vi "Forebrain.vi"() -> ()   [LabVIEW 2012]
doc: "This VI contrains the Forebrain within the Olin Robot Architecture. It must be run first to load the appropriate mission definition files. It contains a finite state machine built around a tabbed Operator interface that will guide an operator through the startup, run shutdown mission sequence. After running it, run the Midbrain and Hindbrain VIS."
panel:
  in  "Lidar cutoff":dbl
  in  "behavior weights":i8[](array[numeric])=[0, 1, 0]
  in  "Follow right?":bool
  in  "Lider good scale mult":dbl=0.0125
  in  "Lider good scale add":dbl
  in  "Lider speed scale add":dbl
  in  "Lider speed scale mult":dbl=0.0175
  in  "IR scaling div":dbl=150.0
  in  "IR Following Distance":i32=300
  out "Ir distance":i16
  in  "Manual Override":bool=TRUE
  out "Send String for AutoMode":string="$B^"
  in  "Soft E-Stop":bool
  out "NXT String Received":string
  out "return count":u32
  out "error out":errorcluster
  in  "error in 2":errorcluster
  out "Desired \nVelocity":i16=5
  out "Local\nHeading":i16=90
  out "Ycurrent":dbl format="%#_3g"
  out "Xcurrent":dbl format="%#_3g"
  out "Ystart":dbl
  out "Xstart":dbl
  in  "error in":errorcluster
  out "Robot Live":bool
  in  "E-Stop":bool
  in  "Tab":T1(tab)
  out "MissionTime (Min)":dbl(knob) scale=0.0..10.0
  out "LidarDist":i16
  out "IR Index":i32
  out "BatteryLevel":dbl(slide) scale=6.0..9.0
  out "String Received":string
  out "Send String":string="$B^"
  in  "VISA resource name":refnum<visa-resource-name>="COM6"
  in  "Mode":i16 min=0 max=99 step=1
  in  "Desired Vel":i16(slide)=7 scale=0.0..14.0
  in  "Local Head":i16(slide)=7 scale=0.0..14.0
  out "StartMissionMap":picture
  out "MapDARCheck":picture
  in  "RunRobot":bool
  in  "Tug letter":string="G"
  out "Tug X":i32
  out "Tug Y":i32
  out "Tug H":i32
  out "BS Time Out?":bool
  out "Buoy locations":cluster{"regular expression":string, i32, i32}[](array[cluster])
  out "Valid ?":bool
  out "Battery\nVolts":i16
  out "Base Station data rec'd":string
  out "udp rate":bool
  out "CollisionWarning":bool
  out "DebugMapDAR":picture
  in  "MapDAR Control":T2={"NumberOfBeams"=180, "SensorRange"=500.0, "Noise (0.1 to 1)"=0.0} {"Noise (0.1 to 1)" min=0.0 max=1.0 step=0.1; "SensorRange" min=500.0 max=1500.0 step=100.0; "NumberOfBeams" min=36 max=360 step=2}
  out "MapDAR Data (r:pixel b:degrees)":cluster{"Range":dbl, "Bearing":dbl}[](array[cluster])
  in  "Stop DebugSENSE":bool
  out "MissionMap":picture
  out "Tug position":T3
  out "initialized MDF":T4(array[cluster])
  out "Way Point Index":i32
  out "InitialWaypoint":cluster{"X":i16, "Y":i16}
  in  "Pen Color":u32(colorbox)=15671808
  in  "Select Pen Attributes":T5={"Width"=1, "Style"=enum."Solid"}
  out "Draw??":bool
  in  "WhereAmI?FromBase":T6
  out "(xr,yr)":cluster{"X":dbl, "Y":dbl}
  in  "RobotPosition":T3 {"xrobot" min=0.0 max=1177.0 step=10.0; "yrobot" min=0.0 max=850.0 step=10.0; "heading" min=0.0 max=7.0 step=0.1}
  out "MDF_Original":T4(array[cluster])
  out "WhatAroundMeMap?":cluster{"T":dbl, "Range":dbl, "Bearing":dbl}[](array[cluster])
  out "WayPointAct":dbl[](array[numeric])
  out "SteerAngle":dbl
  out "MissionDefFile":picture
  out "MDF":T4(array[cluster])
  in  "Select Your Behavior":T7(ring)
  out "No. of Waypoints":i32
  in  "Exit Planning":bool
  in  "BoatSpeed for Leg":dbl(slide)=8.0 min=-9.0 max=9.0 step=1.0 scale=0.0..14.0
  out "BuildMDF":bool
  out "WayPoint Position":cluster{"X":i32, "Y":i32}
  in  "Upper Midbrain Active":bool
  out "Send String to NXT":string="$B^"
  in  "Behavior Command":T7(ring)
  out "CollisionLight":bool
  out "Where? Manual":T6
  out "ActManual":bool
  in  "Manual Heading":i16(knob) min=0 max=14 step=1
  out "MWhat?":bool
  out "Where? 2":bool
  out "How? 2":bool
  in  "ManualModeStop":bool
  out "ManualModeMapDAR":picture
  out "ManualMissionMap":picture
  out "Battery":dbl(slide) scale=0.0..8.0
  in  "Manual Vel":dbl(slide) min=0.0 max=14.0 step=1.0 scale=0.0..14.0
  out "MissionTime":dbl(knob) scale=0.0..10.0
  out "Heading":cluster{dbl, dbl}(knob)={0.0, 34.390870865624734} scale=180.0..-179.0 scale format="%#_3g"
  out "Speed":i16(knob) scale=-6.0..6.0
  out "Current Behavior":T7(ring)
  out "Robot Position":cluster{"X":dbl, "Y":dbl} {"X" format="%#_3g"; "Y" format="%#_3g"}
  out "Ready":bool
  in  "Pause":bool
  in  "Rerun MDF":bool
  out "CollisionLight 2":bool
  out "Act":bool
  out "Neo-C":bool
  out "How?":bool
  out "What?":bool
  out "A Heading":cluster{dbl, dbl}(knob)={0.0, 34.390870865624734} scale=180.0..-180.0
  out "A Speed":dbl(knob) scale=-9.0..9.0
  out "AutoBattery":dbl(slide) scale=0.0..8.0
  out "AutoModeLIDAR":picture
  out "AutoMissionMap":picture
  in  "RunAutoMode":bool
  out "MissionTimeAuto":dbl(knob) scale=0.0..60.0
  out "Where?":bool
  # "To run\nrobot,\nclick\narrow\nabove\n\nRun Robot button must be on"
  # "Operation Directions\n\n1)Click on Startup&\nShutdown tab.\n2) Click on Run \nArrow on menubar.\nRun Forebrain,\nvis from the project\nexplorer.\n3) Select a mssion \nmap file when asked.\n4) Check robot is \nfully operational on\nStartup tab.\n5) Debug with debug\ntabs as required.\n6) Select ManualMode\ntab and test drive \nrobot.\n7) Select PlanMission\ntab and set up \nmission.\n8) Go to AutoMode\ntab and run mission."
  # "Turns off drive\nmotors"
  # "The Tweakers Box"
  # "Enter Olin Test  Pool"
  # "Xbee Com Port"
  # "xBee\"Send String\" (mode, desired velocity, local heading)"
  # "(Type in Tug Letter  L T G P  (look at boat cradle)"
  # "Should be on to\nrun"
  # "BoatG,X,Y,H,BoatT,X,Y,H,BoatP,X,Y.H,BoatL,X,Y,H,BuoyA,X,Y,BuoyB,X,Y,BuoyC,X,Y,BuoyD,X,Y,Time(hours,Min,Sec)"
  # "To stop  program \nturn off here"
  # "Use this tab\nto explore\nLIDAR\ndata and \noperation"
  # "Set\nNumberOfBeams\nSensorRange\nNoise\nto\nview\nsimulated\nsensor\ndata"
  # "Turn Debug Sim \nto leave this\ntab--->"
  # "This tab will auto\nreturn to Startup \nin 2 seconds"
  # "Clean up interface and make more useful for debugging behaviors"
  # "Build out interface and make more useful for debugging act"
  # "This tab will auto\nreturn to Startup \nin 2 seconds"
  # "Directions:\n1) Select Robot Behavior for each mission leg.\n2) Select Robot Speed for leg.\n3) Click on robots current location for first waypoint.\n4) Hold down button and drag to next\nwaypoint. Click on next leg waypoint.\n5) Hold mouse button down and drag to \nnext waypoint. \n6) Click on next waypoint. Repeat for full mission.\n7) MDF will store up to 20 waypoints."
  # "Remember to\nset boat\nleg speed !"
  # "Please Adjust Scroll Barrs in Tug Off Mode to Prevent  Extra Lines Being Drawn"
  # "\"Send String\" (mode, desired velocity, local heading)"
  # "Press to stop and return to StartUp"
  # "Open MidBrain\nArbiter to see\nBrain Waves"
  # "AutoMode\nAutomatically \nReturns to \nStartUp Mode"
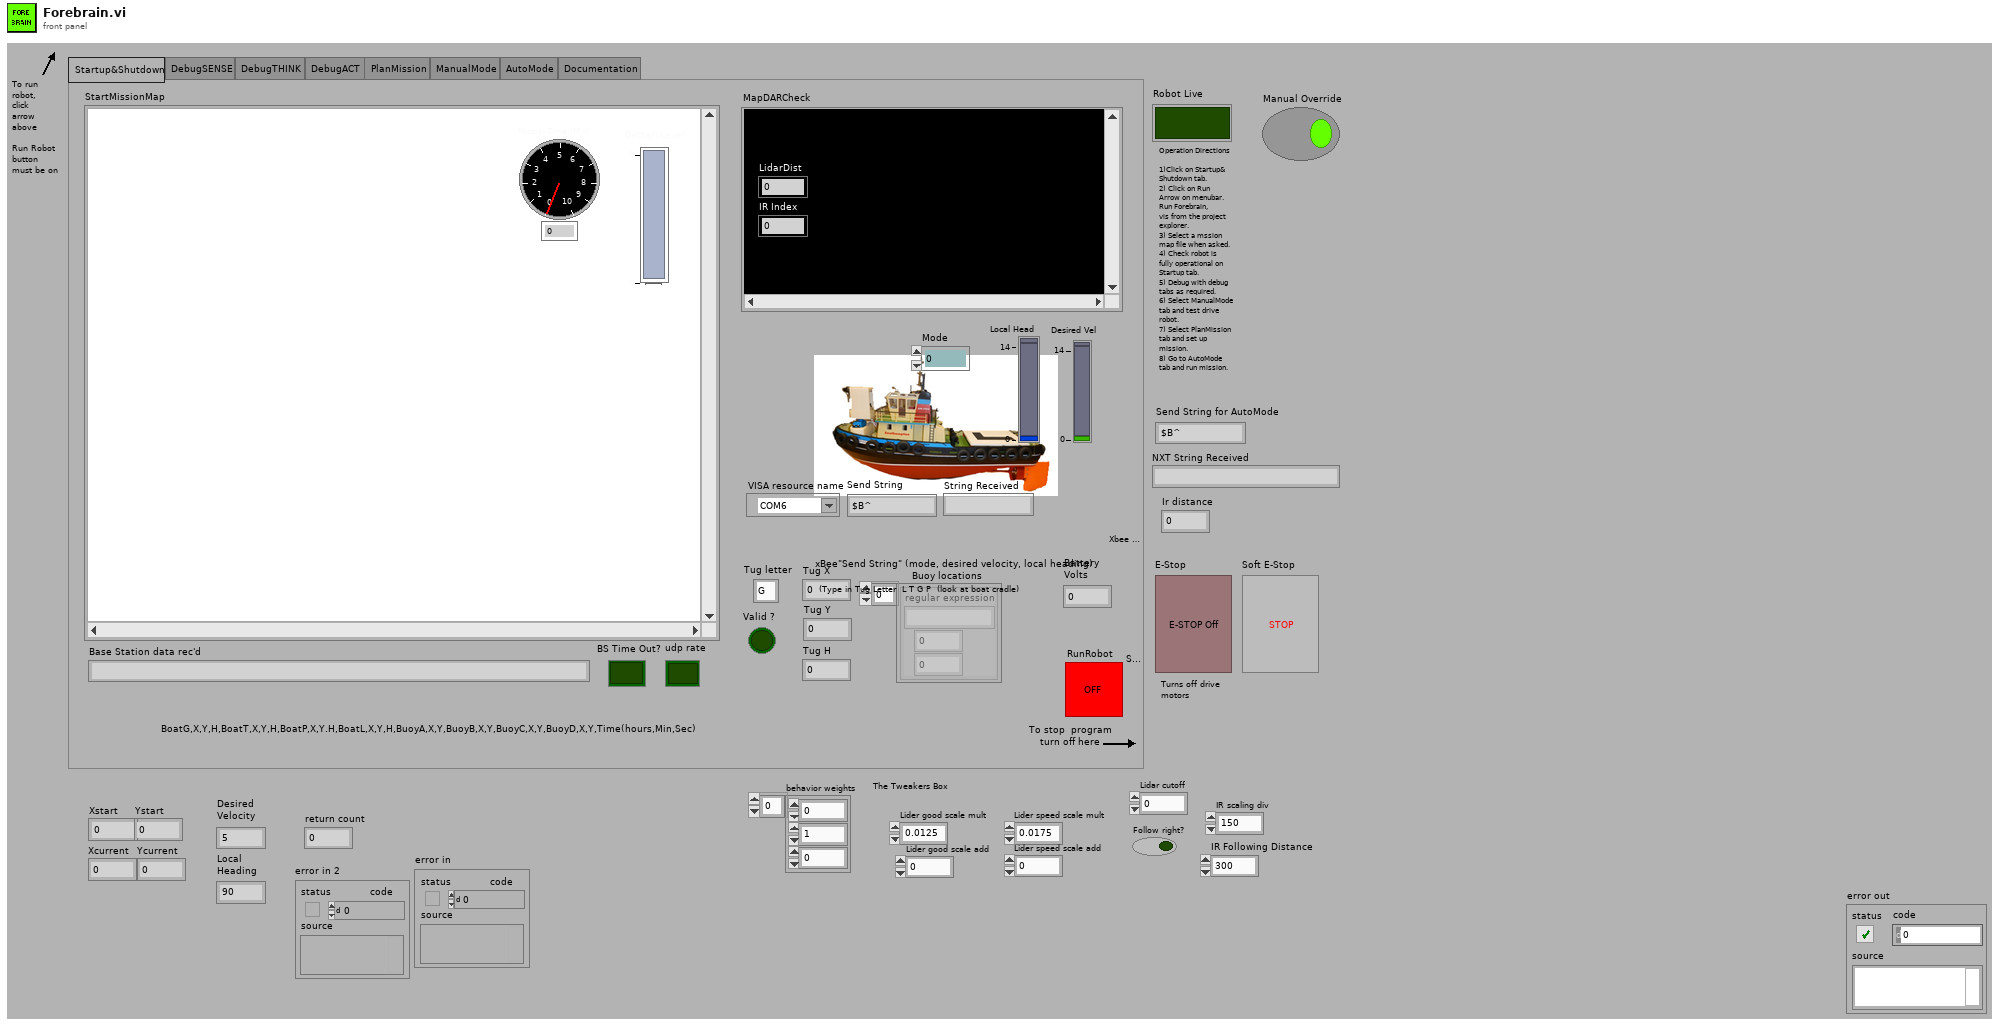
[diagram p1: front panel]
types:
  T1 = enum32{"Startup&Shutdown", "DebugSENSE", "DebugTHINK", "DebugACT", "PlanMission", "ManualMode", "AutoMode", "Documentation"}
  T2 = cluster{"NumberOfBeams":i32, "SensorRange":dbl, "Noise (0.1 to 1)":dbl}
  T3 = cluster{"xrobot":dbl, "yrobot":dbl, "heading":dbl}
  T4 = cluster{"Status":enum16{"Past", "Current", "Future"}, "x":dbl, "y":dbl, "z":dbl, "Vel":dbl, "Dwell Time":dbl, "BehCom":enum16{"Tug Off", "Manual Mode", "Goto WayPoint", "Back Up", "Circle", "Left Wall Follow", "Right Wall Follow", "Hunt"}, "Expand1":dbl, "Expand2":dbl, "Expand3":dbl}[]
  T5 = cluster{"Width":u16, "Style":enum32{"Solid", "Dash", "Dot", "DashDot", "DashDotDot"}}
  T6 = cluster{"T":dbl, "X":dbl, "Y":dbl, "Direction":dbl}
  T7 = enum16{"Tug Off", "Manual Mode", "Goto WayPoint", "Back Up", "Circle", "Left Wall Follow", "Right Wall Follow", "Hunt"}
  T8 = cluster{"VelCom":dbl, "BehCom":enum16{"OpenFieldTransit", "P-WallFollow", "S-WallFollow", "LaneFollow", "ManualMode"}}
  T9 = typedef "IMAQ Image.ctl" = refnum<image>
  T10 = typedef "imagedata.ctl" = cluster{"image type":i32, "image depth":i32, "image":u8[], "mask":u8[], "colors":u32[], "Rectangle":cluster{"left":i16, "top":i16, "right":i16, "bottom":i16}}
  T11 = cluster{"Status":enum16{"Past", "Current", "Future"}, "x":dbl, "y":dbl, "z":dbl, "Vel":dbl, "Dwell Time":dbl, "BehCom":enum16{"Tug Off", "Manual Mode", "Goto WayPoint", "Back Up", "Circle", "Left Wall Follow", "Right Wall Follow", "Hunt"}, "Expand1":dbl, "Expand2":dbl, "Expand3":dbl}
  T12 = typedef "LVMouseTypeDef.ctl" = cluster{"Mouse Position":cluster{"X":i32, "Y":i32}, "Mouse Modifiers":cluster{"Button Down":bool, "Shift Mod":bool, "Menu Mod":bool, "Option Mod":bool}}
  T13 = cluster{"regular expression":string, i32, i32, i32}
  T14 = cluster{"Lider good scale mult":dbl, "Lider good scale add":dbl, "Lider speed scale mult":dbl, "Lider speed scale add":dbl, "Follow right?":bool, "IR Following Distance":i32, "IR scaling div":dbl, "Lidar cutoff":dbl}
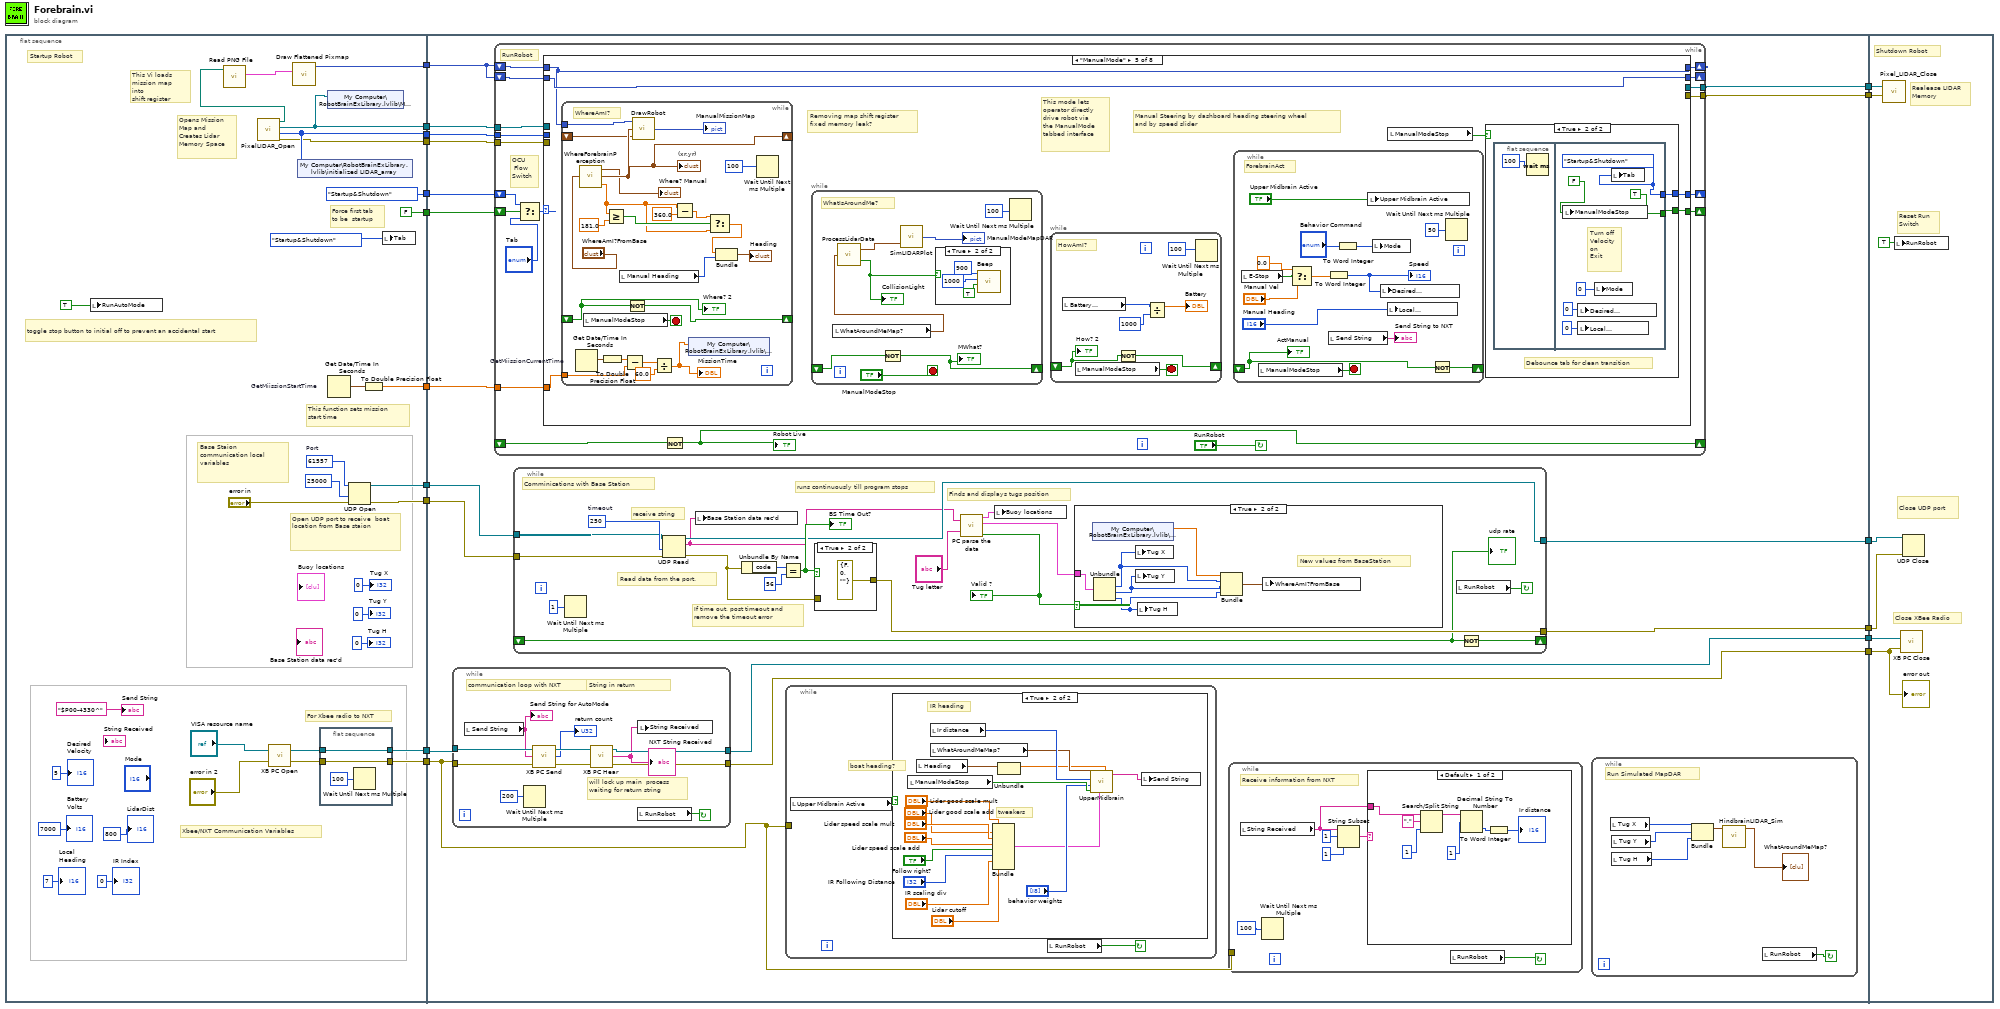
[diagram p0: block diagram]
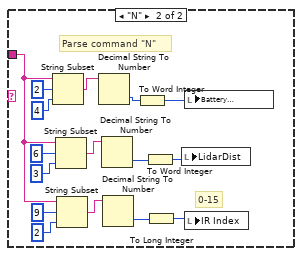
[diagram p2: hidden frame]
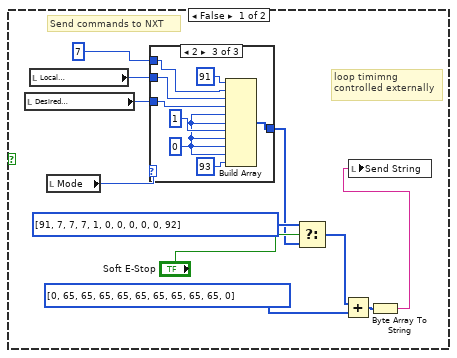
[diagram p3: hidden frame]
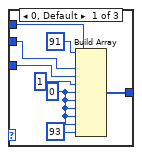
[diagram p4: hidden frame]
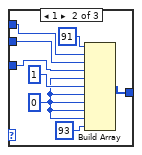
[diagram p5: hidden frame]
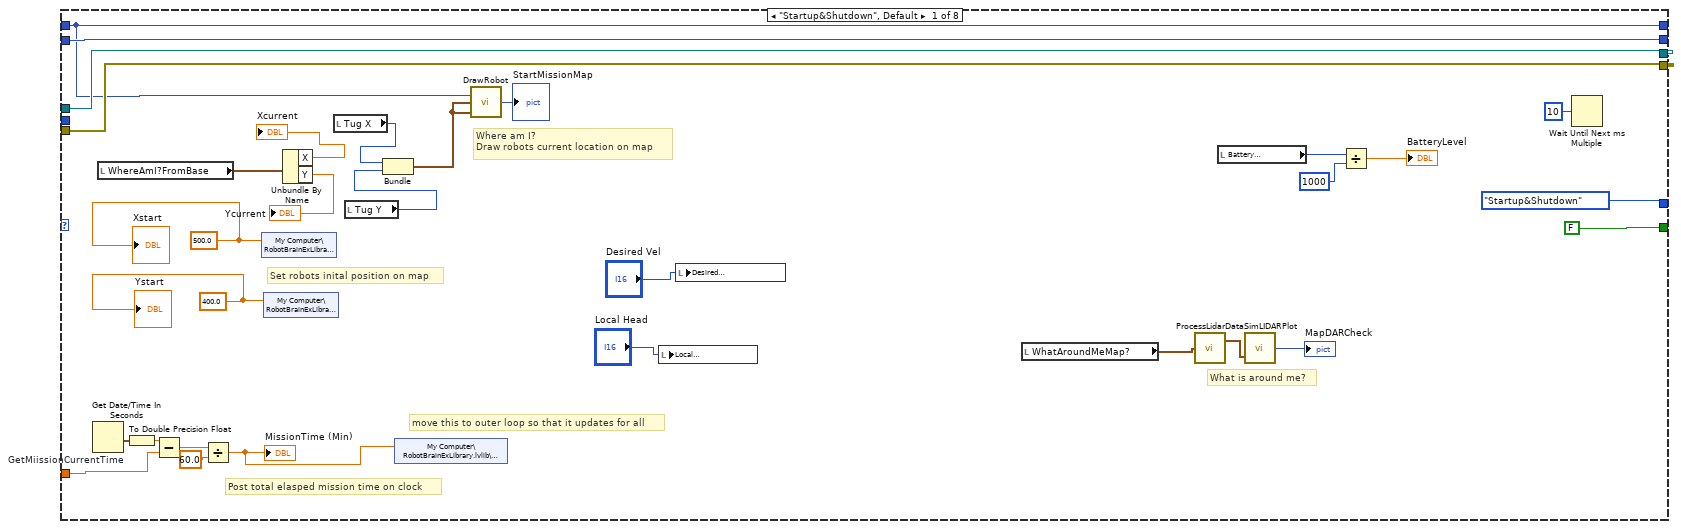
[diagram p8: hidden frame]
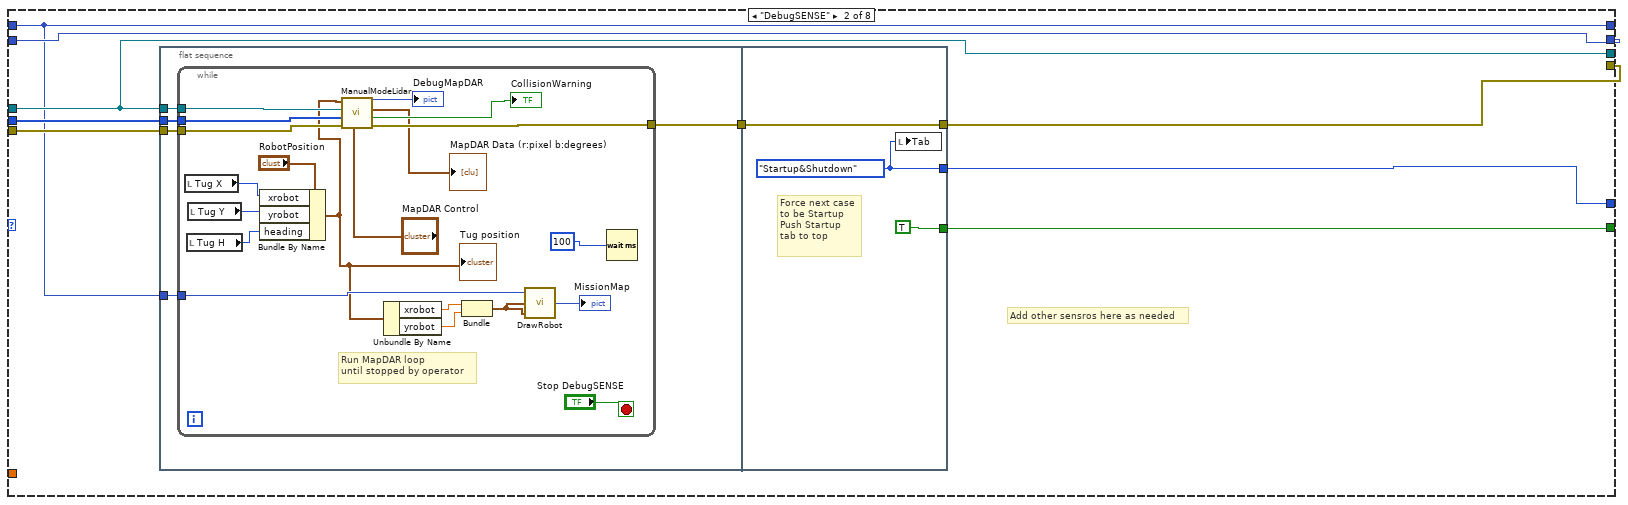
[diagram p9: hidden frame]
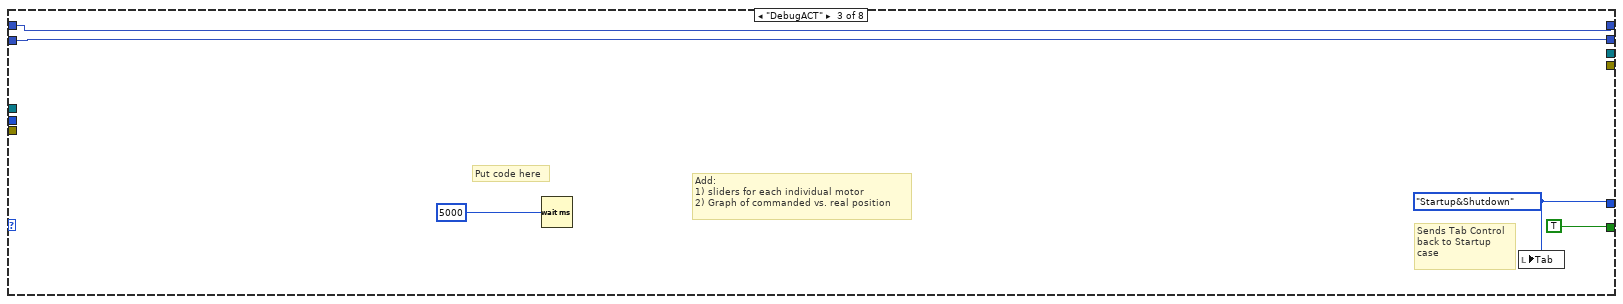
[diagram p10: hidden frame]
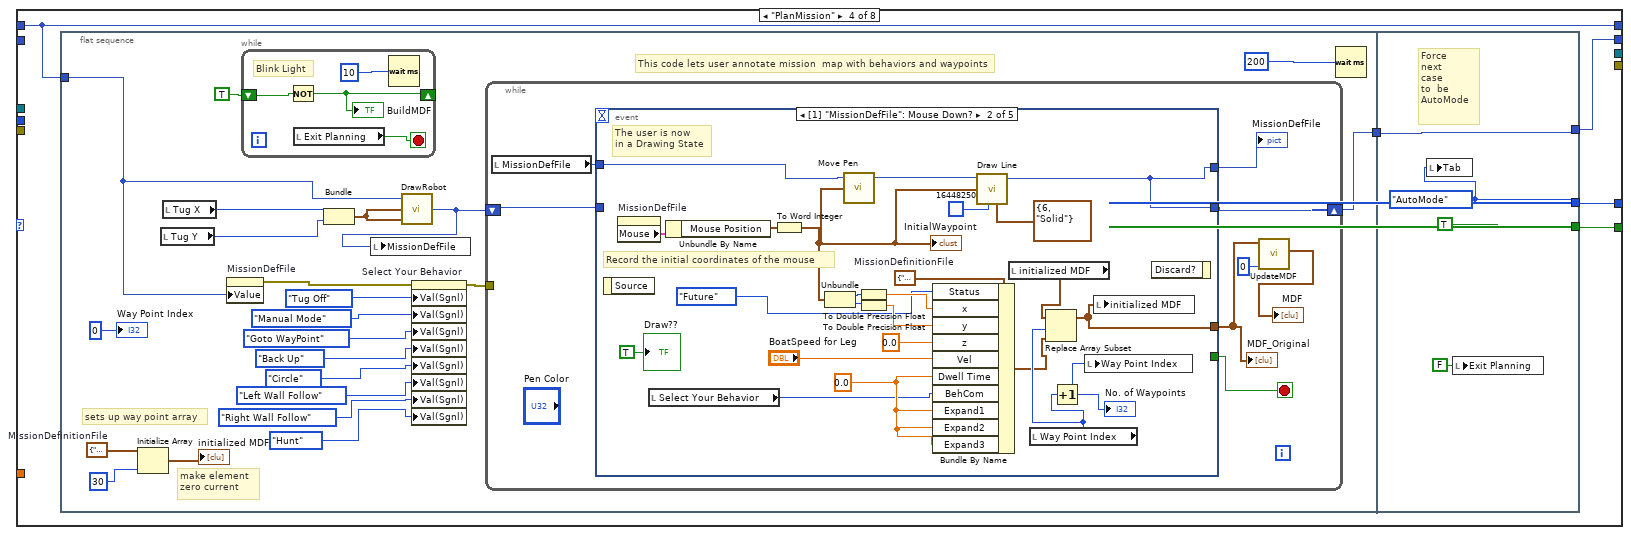
[diagram p11: hidden frame]
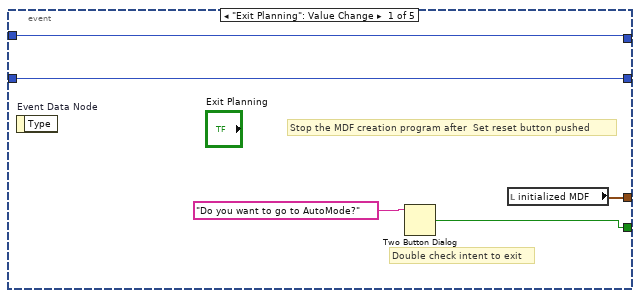
[diagram p12: hidden frame]
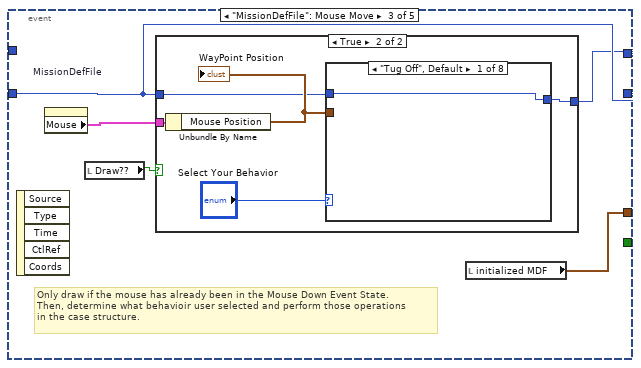
[diagram p13: hidden frame]
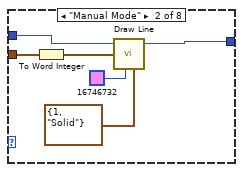
[diagram p15: hidden frame]
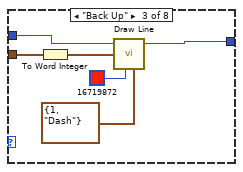
[diagram p16: hidden frame]
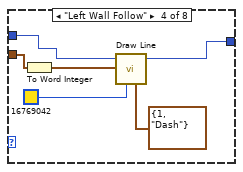
[diagram p17: hidden frame]
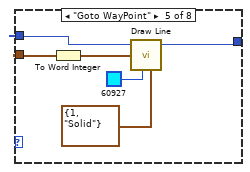
[diagram p18: hidden frame]
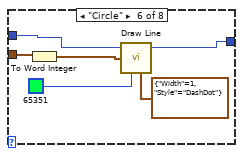
[diagram p19: hidden frame]
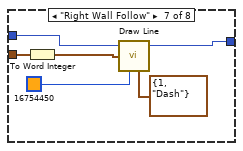
[diagram p20: hidden frame]
diagram:
  n1 = flat-sequence {
    tunnel: [w48] -> w17
    tunnel: [w47] -> w16
    tunnel: [w44] -> w15
    tunnel: [w46] -> w14
    tunnel: [w45] -> w13
    tunnel: [FALSE ("RunAutoMode")] -> w10
    tunnel: [T1."Startup&Shutdown" ("Tab")] -> w9
    tunnel: [w31] -> w8
    tunnel: [w30] -> w7
    tunnel: [w19] -> w6
    tunnel: [w18] -> w5
    tunnel: w17 -> [w69]
    tunnel: w16 -> [w68]
    tunnel: w15 -> [w67]
    tunnel: w14 -> [w66]
    tunnel: w13 -> [w65]
    tunnel: [w64] -> w12
    tunnel: [w63] -> w11
    tunnel: w10 -> [w62]
    tunnel: w9 -> [w61]
    tunnel: w8 -> [w56]
    tunnel: w7 -> [w55]
    tunnel: w6 -> [w60]
    tunnel: w5 -> [w57]
    tunnel: [w59] -> w4
    tunnel: [w58] -> w3
    tunnel: [w54] -> w2
    tunnel: [w53] -> w1
    tunnel: w12 -> [w639]
    tunnel: w11 -> [w638]
    tunnel: w4 -> [w637]
    tunnel: w3 -> [w636]
    tunnel: w2 -> [w635]
    tunnel: w1 -> [w634]
    frame #0 {
      w37 = u16 61557  # Port
      # "For Xbee radio to NXT"
      # "Xbee/NXT Communication Variables"
      # "Base Staion communication local variables"
      # "Open UDP port to receive  boat location from Base staion"
      # "Force first tab\nto be  startup"
      # "toggle stop button to initial off to prevent an accidental start"
      # "Opens Mission\nMap and\nCreates Lidar\nMemory Space"
      # "This function sets mission \nstart time"
      # "This Vi loads\nmission map into \nshift register"
      # "Startup Robot"
      n2 = local write "RunAutoMode"(TRUE ("RunAutoMode")) -> ()
      n3 = call "PixelLIDAR_Open.vi"() -> ("error out"=w45:errorcluster, "initialized LIDAR\narray"=w46:i32[], "MDF Image"=w44:T9, "MissionMap"=w39:path)  [unwired: 2 in]
      n4 = call <vilib>:"Read PNG File.vi"("path to PNG file"=w39) -> ("image data"=w38:T10)  [unwired: 8 in, 2 out]
      n5 = call "XB PC Open.vi"("error in (no error)"="error in 2", "VISA resource name"="VISA resource name") -> ("error out"=w22:errorcluster, "VISA resource name out"=w23:refnum<visa-resource-name>)
      n6 = call <vilib>:"Draw Flattened Pixmap.vi"("image data"=w38) -> ("new picture"=w47:picture)  [unwired: 8 in]
      n7 = shared-variable "My Computer\\RobotBrainExLibrary.lvlib\\initialized LIDAR_array"(w46) -> ()  [unwired: 1 in, 1 out]
      n8 = flat-sequence {
        tunnel: w23 -> [w50]
        tunnel: w22 -> [w51]
        tunnel: [w51] -> w18
        tunnel: [w50] -> w19
        frame #0 {
          n9 = Wait Until Next ms Multiple(millisecond multiple=u32 100) -> ()  [unwired: 1 out]
        }
      }
      n10 = shared-variable "My Computer\\RobotBrainExLibrary.lvlib\\MDF Image"(w44) -> ()  [unwired: 1 in, 1 out]
      n11 = Get Date/Time In Seconds "GetMiissionStartTime"() -> (seconds since 1Jan1904=w49:timestamp)
      n12 = UDP Open(8:"error in", 9:25000 ("timeout ms (25000)"), 11:w37) -> (port=w31:refnum<k16>, 0:w30:errorcluster)  [unwired: 2 in, 1 out]
      n13 = To Double Precision Float(number=w49) -> (double precision float=w48:dbl)
      n14 = local write "Tab"(T1."Startup&Shutdown" ("Tab")) -> ()
      "Tug X" <- 0 ("Tug X")
      "Tug Y" <- 0 ("Tug Y")
      "Tug H" <- 0 ("Tug H")
      "Battery\nVolts" <- i16 7000 ("Battery\nVolts")
      "LidarDist" <- i16 800 ("Dist")
      "IR Index" <- 0 ("IR Index")
      "Local\nHeading" <- i16 7 ("Local\nHeading")
      "Desired \nVelocity" <- i16 5 ("Desired \nVelocity")
      "Send String" <- "$P00-4330^"
    }
    frame #1 {
      n15 = while {
        tunnel: w60 -> [w168]
        tunnel: w57 -> [w167]
        tunnel: [w164] -> w58
        tunnel: [w163] -> w59
        stop <- w162 continue-if-true
        # "will lock up main  process\nwaiting for return string"
        # "communication loop with NXT"
        # "send a string to the NXT and receive a String in return"
        n16 = local read "Send String"() -> (w160:string)
        "Send String for AutoMode" <- w160
        n17 = Wait Until Next ms Multiple(millisecond multiple=u32 200) -> ()  [unwired: 1 out]
        n18 = call "XB PC Send.vi"("error in (no error)"=w167, "String"=w160, "VISA resource name"=w168) -> ("error out"=w166:errorcluster, "return count"=→"return count":u32, "VISA resource name out"=w165:refnum<visa-resource-name>)
        n19 = call "XB PC Hear.vi"("VISA resource name"=w165, "error in (no error)"=w166) -> ("VISA resource name out"=w163:refnum<visa-resource-name>, "String Received"=w159:string, "error out"=w164:errorcluster)
        "NXT String Received" <- w159
        n20 = local read "RunRobot"() -> (w162:bool)
        n21 = local write "String Received"(w159) -> ()
      }
      n22 = while {
        shift-right: [w195] -> _
        shift-left: _ -> [w212]
        shift-right: [w211] -> _
        shift-left: w61 -> [w210]
        shift-right: [w207] -> _
        shift-left: w62 -> [w206]
        tunnel: w69 -> [w205]
        shift-right: [w203] -> _
        shift-left: w68 -> [w204]
        shift-right: [w201] -> _
        shift-left: w68 -> [w202]
        tunnel: w67 -> [w200]
        tunnel: w66 -> [w199]
        tunnel: w65 -> [w198]
        tunnel: [w197] -> w64
        tunnel: [w196] -> w63
        stop <- "RunRobot" continue-if-true
        # "RunRobot"
        # "OCU\n Flow\nSwitch"
        n23 = Select(t=w210, s=w206, f="Tab") -> (s? t:f=w208:T1)
        n24 = case shown="\"ManualMode\"" w208 {
          selector: w208 -> [_ _ _ _ _ w532 _ _]
          tunnel: [T1."Startup&Shutdown" ("Tab") w248 w283 w290 w457 w533 T1."Startup&Shutdown" ("Tab") w632] -> w211
          tunnel: [FALSE ("s") w247 TRUE ("s") w289 w458 w531 FALSE ("s") TRUE ("s")] -> w207
          tunnel: w205 -> [w237 _ _ _ w455 w529 _ _]
          tunnel: w204 -> [w230 w244 w282 w286 w453 w526 w625 w630]
          tunnel: [w230 w244 w282 w286 w453 w526 w625 w630] -> w203
          tunnel: w202 -> [w236 w245 w281 _ w454 w528 w624 w629]
          tunnel: [w236 w245 w281 w287 w454 w528 w624 w629] -> w201
          tunnel: w200 -> [w235 w246 _ _ _ _ _ _]
          tunnel: w199 -> [_ w252 _ _ _ _ _ _]
          tunnel: w198 -> [w234 w251 _ _ _ _ _ _]
          tunnel: [w235 w246 _ _ _ _ _ _] -> w197
          tunnel: [w234 w250 _ _ _ _ _ _] -> w196
          frame "Startup&Shutdown", Default {
            w225 = 400.0 ("Ystart")
            w226 = 500.0 ("Xstart")
            # "move this to outer loop so that it updates for all"
            # "Where am I?\nDraw robots current location on map"
            # "Post total elasped mission time on clock"
            # "What is around me?"
            # "Set robots inital position on map"
            n25 = Get Date/Time In Seconds "GetMiissionCurrentTime"() -> (seconds since 1Jan1904=w241:timestamp)
            n26 = local read "WhereAmI?FromBase"() -> (w214:T6)
            n27 = To Double Precision Float(number=w241) -> (double precision float=w240:dbl)
            n28 = Subtract(x=w240, y=w237) -> (x-y=w239:dbl)
            n29 = Divide(x=w239, y=60.0) -> (x/y=w233:dbl)
            "MissionTime (Min)" <- w233
            n30 = shared-variable "My Computer\\RobotBrainExLibrary.lvlib\\Xstart"(w226) -> ()  [unwired: 1 in, 1 out]
            n31 = shared-variable "My Computer\\RobotBrainExLibrary.lvlib\\Ystart"(w225) -> ()  [unwired: 1 in, 1 out]
            n32 = Unbundle By Name(w214) -> ("X"=→"Xcurrent":dbl, "Y"=→"Ycurrent":dbl)
            n33 = local read "Tug X"() -> (w224:i32)
            n34 = local read "Tug Y"() -> (w223:i32)
            n35 = Bundle("Tug X"=w224, "Tug Y"=w223) -> (w229:cluster{"Tug X":i32, "Tug Y":i32})  [unwired: 1 in]
            n36 = shared-variable "My Computer\\RobotBrainExLibrary.lvlib\\MissionTime"(w233) -> ()  [unwired: 1 in, 1 out]
            n37 = call "DrawRobot.vi"("(xr,yr) old"=w229, "(xr,yr) new"=w229, "2D Picture"=w230) -> ("new picture"=→"StartMissionMap":picture)
            n38 = local write "Local\nHeading"("Local Head") -> ()
            n39 = local write "Desired \nVelocity"("Desired Vel") -> ()
            n40 = local read "WhatAroundMeMap?"() -> (w215:cluster{"T":dbl, "Range":dbl, "Bearing":dbl}[])
            n41 = call "ProcessLidarData.vi"("WhatAroundMe?MM"=w215) -> ("data array [mag, phase (deg)]"=w231:cluster{"magnitude":dbl, "phase":dbl}[])  [unwired: 1 out]
            n42 = local read "Battery\nVolts"() -> (w220:i16)
            n43 = call "SimLIDARPlot.vi"("data array [mag, phase (deg)]"=w231) -> ("SONAR"=→"MapDARCheck":picture)  [unwired: 1 in]
            n44 = Divide(x=w220, y=i16 1000) -> (x/y=→"BatteryLevel":dbl)
            n45 = Wait Until Next ms Multiple(millisecond multiple=u32 10) -> ()  [unwired: 1 out]
            "Xstart" <- w226
            "Ystart" <- w225
          }
          frame "DebugSENSE" {
            # "Add other sensros here as needed"
            n46 = flat-sequence {
              tunnel: w252 -> [w257]
              tunnel: w251 -> [w256]
              tunnel: w246 -> [w255]
              tunnel: [w254] -> w249
              tunnel: w244 -> [w253]
              tunnel: [w280] -> w250
              tunnel: w249 -> [w280]
              tunnel: [w279] -> w248
              tunnel: [TRUE ("s")] -> w247
              frame #0 {
                n47 = while {
                  tunnel: w257 -> [w277]
                  tunnel: w256 -> [w276]
                  tunnel: w255 -> [w275]
                  tunnel: [w274] -> w254
                  tunnel: w253 -> [w268]
                  stop <- "Stop DebugSENSE" stop-if-true
                  # "Run MapDAR loop\nuntil stopped by operator"
                  n48 = local read "Tug X"() -> (w262:i32)
                  n49 = local read "Tug H"() -> (w263:i32)
                  n50 = local read "Tug Y"() -> (w261:i32)
                  n51 = Bundle By Name(cluster="RobotPosition", "xrobot"=w262, "yrobot"=w261, "heading"=w263) -> (w259:T3)
                  "Tug position" <- w259
                  n52 = call "ManualModeLidar.vi"("LIDARControl"="MapDAR Control", "error in"=w276, "initialized \nsonar ray\narray"=w277, "MDF Image"=w275, "SubPosition"=w259) -> ("error out"=w274:errorcluster, "Collision\nWarning"=→"CollisionWarning":bool, "LIDAR Data (r:pixel b:degrees)"=→"MapDAR Data (r:pixel b:degrees)":cluster{"Range":dbl, "Bearing":dbl}[], "LIDAR"=→"DebugMapDAR":picture)  [unwired: 1 in]
                  n53 = Unbundle By Name(w259) -> ("xrobot"=w266:dbl, "yrobot"=w265:dbl)
                  n54 = Bundle("xrobot"=w266, "yrobot"=w265) -> (w258:cluster{"xrobot":dbl, "yrobot":dbl})  [unwired: 1 in]
                  n55 = call "DrawRobot.vi"("(xr,yr) old"=w258, "(xr,yr) new"=w258, "2D Picture"=w268) -> ("new picture"=→"MissionMap":picture)
                  n56 = Wait (ms)(milliseconds to wait=u32 100) -> ()  [unwired: 1 out]
                }
              }
              frame #1 {
                w279 = T1."Startup&Shutdown" ("Tab")
                # "Force next case\nto be Startup\nPush Startup\ntab to top"
                n57 = local write "Tab"(w279) -> ()
              }
            }
          }
          frame "DebugACT" {
            w283 = T1."Startup&Shutdown" ("Tab")
            # "Add:\n1) sliders for each individual motor\n2) Graph of commanded vs. real position"
            # "Put code here"
            # "Sends Tab Control\nback to Startup\ncase"
            n58 = Wait (ms)(milliseconds to wait=u32 5000) -> ()  [unwired: 1 out]
            n59 = local write "Tab"(w283) -> ()
          }
          frame "PlanMission" {
            n60 = flat-sequence {
              tunnel: [w311] -> w288
              tunnel: w286 -> [w304]
              tunnel: [w451] -> w290
              tunnel: [TRUE ("s")] -> w289
              tunnel: w288 -> [w450]
              tunnel: [w450] -> w287
              frame #0 {
                w302 = T11 {"Status"=enum."Future", "x"=0.0, "y"=0.0, "z"=0.0, "Vel"=0.0, "Dwell Time"=0.0, "BehCom"=enum."Tug Off", "Expand1"=0.0, "Expand2"=0.0, "Expand3"=0.0}  # MissionDefinitionFile
                # "make element \nzero current"
                # "sets up way point array"
                # "This code lets user annotate mission  map with behaviors and waypoints"
                n61 = Initialize Array ("Initialize WaypointArray")(w302, 30 ("dimension size")) -> (→"initialized MDF":T4)
                n62 = local read "Tug Y"() -> (w299:i32)
                n63 = local read "Tug X"() -> (w300:i32)
                n64 = property on="MissionDefFile" class="Pict"("Value"=w304) -> (error out=w309:errorcluster)  [unwired: 2 in, 1 out]
                n65 = while {
                  shift-right: [w315] -> _
                  shift-left: TRUE -> [w316]
                  stop <- w314 stop-if-true
                  # "Blink Light"
                  n66 = Not(x=w316) -> (.not. x?=w315:bool)
                  "BuildMDF" <- w315
                  n67 = local read "Exit Planning"() -> (w314:bool)
                  n68 = Wait (ms)(milliseconds to wait=u32 10) -> ()  [unwired: 1 out]
                }
                n69 = Bundle("Tug X"=w300, "Tug Y"=w299) -> (w305:cluster{"Tug X":i32, "Tug Y":i32})  [unwired: 1 in]
                n70 = call "DrawRobot.vi"("(xr,yr) old"=w305, "(xr,yr) new"=w305, "2D Picture"=w304) -> ("new picture"=w303:picture)
                n71 = local write "MissionDefFile"(w303) -> ()
                n72 = property on="Select Your Behavior" class="Enum (strict)"(error in=w309, "Val(Sgnl)"=T7."Tug Off" ("Value (Signaling)"), "Val(Sgnl)"=T7."Manual Mode" ("Value (Signaling)"), "Val(Sgnl)"=T7."Goto WayPoint" ("Value (Signaling)"), "Val(Sgnl)"=T7."Back Up" ("Value (Signaling)"), "Val(Sgnl)"=T7."Circle" ("Value (Signaling)"), "Val(Sgnl)"=T7."Left Wall Follow" ("Value (Signaling)"), "Val(Sgnl)"=T7."Right Wall Follow" ("Value (Signaling)"), "Val(Sgnl)"=T7."Hunt" ("Value (Signaling)")) -> (error out=w310:errorcluster)  [unwired: 1 in, 1 out]
                n73 = while {
                  shift-right: [w323] -> w311
                  shift-left: w303 -> [w324]
                  tunnel: w310 -> [_]
                  stop <- w322 stop-if-true
                  n74 = local read "MissionDefFile"() -> (w321:picture)
                  n75 = event shown="[1] \"MissionDefFile\": Mouse Down?" {
                    selector: _ -> [_ _ _ _ _]
                    dyn-events: _ -> [_ _ _ _ _]
                    timeout: _ -> [_ _ _ _ _]
                    tunnel: [w327 w335 w355 w408 w446] -> w323
                    tunnel: w324 -> [w327 _ w355 w408 _]
                    tunnel: [w328 _ _ _ _] -> w322
                    tunnel: [w326 w350 w356 w410 w447] -> w318
                    tunnel: w321 -> [w325 w336 _ w409 w446]
                    tunnel: [w325 w335 w354 w409 w446] -> w320
                    event "Exit Planning": Value Change {
                      # "Double check intent to exit"
                      # "Stop the MDF creation program after  Set reset button pushed"
                      n76 = event-data "Event Data Node"() -> ()  [unwired: 1 in, 1 out]
                      n77 = Two Button Dialog(message="Do you want to go to AutoMode?") -> (T button?=w328:bool)  [unwired: 2 in]
                      n78 = local read "initialized MDF"() -> (w326:T4)
                    }
                    event "MissionDefFile": Mouse Down? {
                      w334 = T11 {"Status"=enum."Future", "x"=0.0, "y"=0.0, "z"=0.0, "Vel"=0.0, "Dwell Time"=0.0, "BehCom"=enum."Tug Off", "Expand1"=0.0, "Expand2"=0.0, "Expand3"=0.0}  # MissionDefinitionFile
                      w344 = 0.0 ("Dwell Time")
                      # "Record the initial coordinates of the mouse"
                      # "The user is now\nin a Drawing State"
                      n79 = event-data() -> ()  [unwired: 1 in, 1 out]
                      n80 = property on="MissionDefFile" class="Pict"() -> ("Mouse"=w353:T12)  [unwired: 2 in, 2 out]
                      n81 = local read "Select Your Behavior"() -> (w331:T7)
                      n82 = Unbundle By Name(w353) -> ("Mouse Position"=w351:cluster{"X":i32, "Y":i32})
                      n83 = To Word Integer(number=w351) -> (16bit integer=w339:cluster{"X":i16, "Y":i16})
                      "InitialWaypoint" <- w339
                      n84 = Unbundle(w339) -> ("X"=w348:i16, "Y"=w347:i16)
                      n85 = call <vilib>:"Move Pen.vi"("new position"=w339, "picture"=w336) -> ("new picture"=w340:picture)  [unwired: 3 in]
                      n86 = To Double Precision Float(number=w348) -> (double precision float=w346:dbl)
                      n87 = To Double Precision Float(number=w347) -> (double precision float=w345:dbl)
                      n88 = Bundle By Name(cluster=w334, "Status"=enum16{"Past", "Current", "Future"}."Future", "x"=w346, "y"=w345, "z"=0.0, "Vel"="BoatSpeed for Leg", "Dwell Time"=w344, "BehCom"=w331, "Expand1"=w344, "Expand2"=w344, "Expand3"=w344) -> (w330:T11)
                      n89 = call <vilib>:"Draw Line.vi"("picture"=w340, "end point"=w339, "color(black)"=u32 16448250, "pen"=T5 {"Width"=6, "Style"=enum."Solid"}) -> ("new picture"=w335:picture)  [unwired: 5 in]
                      n90 = local read "initialized MDF"() -> (w349:T4)
                      n91 = local read "Way Point Index"() -> (w332:i32)
                      n92 = Replace Array Subset(array=w349, new element=w330, index=w332) -> (w350:T4)
                      n93 = Increment(x=w332) -> (x+1=w352:i32)
                      "No. of Waypoints" <- w352
                      n94 = local write "Way Point Index"(w352) -> ()
                      n95 = local write "initialized MDF"(w350) -> ()
                      n96 = event-data() -> ()  [unwired: 2 in, 1 out]
                      "Draw??" <- TRUE ("Draw??")
                    }
                    event "MissionDefFile": Mouse Move {
                      # "Only draw if the mouse has already been in the Mouse Down Event State.\nThen, determine what behavioir user selected and perform those operations\nin the case structure."
                      n97 = event-data() -> ()  [unwired: 1 in, 5 out]
                      n98 = property on="MissionDefFile" class="Pict"() -> ("Mouse"=w358:T12)  [unwired: 2 in, 2 out]
                      n99 = local read "Draw??"() -> (w357:bool)
                      n100 = case shown="True" w357 {
                        tunnel: w358 -> [_ w364]
                        tunnel: w355 -> [w359 w360]
                        tunnel: [w359 w361] -> w354
                        frame False {
                        }
                        frame True {
                          n101 = Unbundle By Name(w364) -> ("Mouse Position"=w362:cluster{"X":i32, "Y":i32})
                          "WayPoint Position" <- w362
                          n102 = case shown="\"Tug Off\", Default" "Select Your Behavior" {
                            tunnel: w362 -> [_ w370 w376 w379 w385 w390 w396 w402]
                            tunnel: [w365 w371 w377 w381 w384 w391 w397 w403] -> w361
                            tunnel: w360 -> [w365 w369 w373 w382 w386 w392 w398 w404]
                            frame "Tug Off", Default {
                            }
                            frame "Manual Mode" {
                              n103 = To Word Integer(number=w370) -> (16bit integer=w366:cluster{"X":i16, "Y":i16})
                              n104 = call <vilib>:"Draw Line.vi"("picture"=w369, "end point"=w366, "color(black)"=u32 16746732, "pen"=T5 {"Width"=1, "Style"=enum."Solid"}) -> ("new picture"=w371:picture)  [unwired: 5 in]
                            }
                            frame "Back Up" {
                              n105 = To Word Integer(number=w376) -> (16bit integer=w372:cluster{"X":i16, "Y":i16})
                              n106 = call <vilib>:"Draw Line.vi"("picture"=w373, "end point"=w372, "color(black)"=u32 16719872, "pen"=T5 {"Width"=1, "Style"=enum."Dash"}) -> ("new picture"=w377:picture)  [unwired: 5 in]
                            }
                            frame "Left Wall Follow" {
                              n107 = To Word Integer(number=w379) -> (16bit integer=w380:cluster{"X":i16, "Y":i16})
                              n108 = call <vilib>:"Draw Line.vi"("picture"=w382, "end point"=w380, "color(black)"=u32 16769042, "pen"=T5 {"Width"=1, "Style"=enum."Dash"}) -> ("new picture"=w381:picture)  [unwired: 5 in]
                            }
                            frame "Goto WayPoint" {
                              n109 = To Word Integer(number=w385) -> (16bit integer=w387:cluster{"X":i16, "Y":i16})
                              n110 = call <vilib>:"Draw Line.vi"("picture"=w386, "end point"=w387, "color(black)"=u32 60927, "pen"=T5 {"Width"=1, "Style"=enum."Solid"}) -> ("new picture"=w384:picture)  [unwired: 5 in]
                            }
                            frame "Circle" {
                              n111 = To Word Integer(number=w390) -> (16bit integer=w395:cluster{"X":i16, "Y":i16})
                              n112 = call <vilib>:"Draw Line.vi"("picture"=w392, "end point"=w395, "color(black)"=u32 65351, "pen"=T5 {"Width"=1, "Style"=enum."DashDot"}) -> ("new picture"=w391:picture)  [unwired: 5 in]
                            }
                            frame "Right Wall Follow" {
                              n113 = To Word Integer(number=w396) -> (16bit integer=w401:cluster{"X":i16, "Y":i16})
                              n114 = call <vilib>:"Draw Line.vi"("picture"=w398, "end point"=w401, "color(black)"=u32 16754450, "pen"=T5 {"Width"=1, "Style"=enum."Dash"}) -> ("new picture"=w397:picture)  [unwired: 5 in]
                            }
                            frame "Hunt" {
                              n115 = To Word Integer(number=w402) -> (16bit integer=w405:cluster{"X":i16, "Y":i16})
                              n116 = call <vilib>:"Draw Line.vi"("picture"=w404, "end point"=w405, "color(black)"=u32 16720896, "pen"=T5 {"Width"=1, "Style"=enum."DashDotDot"}) -> ("new picture"=w403:picture)  [unwired: 5 in]
                            }
                          }
                        }
                      }
                      n117 = local read "initialized MDF"() -> (w356:T4)
                    }
                    event "Select Your Behavior": Value Change {
                      # "When the user selects a new operation, we disable certain controls that aren't relevant to\nthe operation that the user is performing."
                      n118 = event-data() -> ("NewVal"=w413:T7)  [unwired: 1 in]
                      n119 = property on="Select Pen Attributes" class="Clust (strict)"() -> ("Controls[]"=w412:refnum<vi>[])  [unwired: 2 in, 2 out]
                      n120 = case shown="\"Manual Mode\"" w413 {
                        tunnel: w412 -> [w417 w418 w422 w426 w430 w434 w438 w442]
                        tunnel: "Select Pen Attributes" -> [_ _ _ _ _ _ _ _]
                        frame "Manual Mode" {
                          # "All attributes are valid for this\noperation."
                          n121 = Index Array "Index Array"(array=w417, index=1) -> (element=w415:refnum<vi>)
                          n122 = property on="Property Node" class="Ctl"(reference=w415, "Disabled"=u8 0) -> ()  [unwired: 1 in, 2 out]
                        }
                        frame "Back Up" {
                          # "All attributes are valid for this\noperation."
                          n123 = Index Array(array=w418, index=1) -> (element=w420:refnum<vi>)
                          n124 = property class="Ctl"(reference=w420, "Disabled"=u8 0) -> ()  [unwired: 1 in, 2 out]
                        }
                        frame "Tug Off" {
                          # "All attributes are valid for this\noperation."
                          n125 = Index Array "Index Array"(array=w422, index=1) -> (element=w424:refnum<vi>)
                          n126 = property on="Property Node" class="Ctl"(reference=w424, "Disabled"=u8 0) -> ()  [unwired: 1 in, 2 out]
                        }
                        frame "Left Wall Follow" {
                          # "All attributes are valid for this\noperation."
                          n127 = Index Array "Index Array"(array=w426, index=1) -> (element=w428:refnum<vi>)
                          n128 = property on="Property Node" class="Ctl"(reference=w428, "Disabled"=u8 0) -> ()  [unwired: 1 in, 2 out]
                        }
                        frame "Goto WayPoint" {
                          # "All attributes are valid for this\noperation."
                          n129 = Index Array "Index Array"(array=w430, index=1) -> (element=w432:refnum<vi>)
                          n130 = property on="Property Node" class="Ctl"(reference=w432, "Disabled"=u8 0) -> ()  [unwired: 1 in, 2 out]
                        }
                        frame "Circle" {
                          # "All attributes are valid for this\noperation."
                          n131 = Index Array "Index Array"(array=w434, index=1) -> (element=w436:refnum<vi>)
                          n132 = property on="Property Node" class="Ctl"(reference=w436, "Disabled"=u8 0) -> ()  [unwired: 1 in, 2 out]
                        }
                        frame "Right Wall Follow" {
                          # "All attributes are valid for this\noperation."
                          n133 = Index Array "Index Array"(array=w438, index=1) -> (element=w440:refnum<vi>)
                          n134 = property on="Property Node" class="Ctl"(reference=w440, "Disabled"=u8 0) -> ()  [unwired: 1 in, 2 out]
                        }
                        frame "Hunt" {
                          # "All attributes are valid for this\noperation."
                          n135 = Index Array "Index Array"(array=w442, index=1) -> (element=w444:refnum<vi>)
                          n136 = property on="Property Node" class="Ctl"(reference=w444, "Disabled"=u8 0) -> ()  [unwired: 1 in, 2 out]
                        }
                      }
                      n137 = local read "initialized MDF"() -> (w410:T4)
                    }
                    event "MissionDefFile": Mouse Up {
                      # "When the user is finished drawing, we complete the operation."
                      # "Finished Drawing"
                      n138 = event-data() -> ()  [unwired: 1 in, 3 out]
                      n139 = local write "Draw??"(FALSE ("Draw??")) -> ()
                      n140 = local read "initialized MDF"() -> (w447:T4)
                    }
                  }
                  "MissionDefFile" <- w320
                  "MDF_Original" <- w318
                  n141 = call "UpdateMDF.vi"("Index"=0, "MDF_In"=w318) -> ("MDF_Out"=→"MDF":T4)  [unwired: 9 in]
                }
                n142 = Wait (ms)(milliseconds to wait=u32 200) -> ()  [unwired: 1 out]
                "Way Point Index" <- 0 ("Boundary Point Index")
              }
              frame #1 {
                w451 = T1."AutoMode" ("Tab")
                # "Force \nnext \ncase\nto  be\nAutoMode"
                n143 = local write "Tab"(w451) -> ()
                n144 = local write "Exit Planning"(FALSE ("Exit Planning")) -> ()
              }
            }
          }
          frame "ManualMode" {
            # "Removing map shift register\nfixed memory leak?"
            # "Manual Steering by dashboard heading steering wheel\nand by speed slider"
            # "This mode lets \noperator directly\ndrive robot via\nthe ManualMode\ntabbed interface"
            n145 = while {
              shift-right: [w481] -> _
              shift-left: _ -> [w480]
              tunnel: w455 -> [w473]
              shift-right: [w470] -> _
              shift-left: _ -> [w469]
              tunnel: w453 -> [w467]
              stop <- w479 stop-if-true
              # "WhereAmI?"
              n146 = Get Date/Time In Seconds "GetMiissionCurrentTime"() -> (seconds since 1Jan1904=w474:timestamp)
              n147 = call "WhereForebrainPerception.vi"("Where? Midbrain"="WhereAmI?FromBase") -> ("Where? Forebrain"=→"Where? Manual":T6, "(xr,yr)"=w470:cluster{"X":dbl, "Y":dbl}, "Direction"=w459:dbl)  [unwired: 3 in, 1 out]
              "(xr,yr)" <- w470
              n148 = local read "ManualModeStop"() -> (w479:bool)
              n149 = To Double Precision Float(number=w474) -> (double precision float=w475:dbl)
              n150 = Greater Or Equal?(x=w459, y=181.0) -> (x >= y?=w464:bool)
              n151 = local read "Manual Heading"() -> (w471:i16)
              n152 = Subtract(x=w475, y=w473) -> (x-y=w476:dbl)
              n153 = Not(x=w480) -> (.not. x?=w481:bool)
              n154 = call "DrawRobot.vi"("(xr,yr) old"=w469, "(xr,yr) new"=w470, "2D Picture"=w467) -> ("new picture"=→"ManualMissionMap":picture)
              n155 = Divide(x=w476, y=60.0) -> (x/y=w478:dbl)
              "MissionTime" <- w478
              n156 = Subtract(x=w459, y=360.0) -> (x-y=w462:dbl)
              n157 = shared-variable "My Computer\\RobotBrainExLibrary.lvlib\\MissionTime"(w478) -> ()  [unwired: 1 in, 1 out]
              n158 = Select(t=w462, s=w464, f=w459) -> (s? t:f=w461:dbl)
              n159 = Bundle("Direction"=w461, "Manual Heading"=w471) -> (→"Heading":cluster{"Direction":dbl, "Manual Heading":i16})  [unwired: 1 in]
              n160 = Wait Until Next ms Multiple(millisecond multiple=u32 100 ("milliseconds to wait")) -> ()  [unwired: 1 out]
              "Where? 2" <- w480
            }
            n161 = while {
              shift-right: [w488] -> _
              shift-left: _ -> [w489]
              stop <- "ManualModeStop" stop-if-true
              # "WhatIsAroundMe?"
              n162 = local read "WhatAroundMeMap?"() -> (w483:cluster{"T":dbl, "Range":dbl, "Bearing":dbl}[])
              n163 = call "ProcessLidarData.vi"("WhatAroundMe?MM"=w483) -> ("Collision"=w484:bool, "data array [mag, phase (deg)]"=w485:cluster{"magnitude":dbl, "phase":dbl}[])
              "CollisionLight" <- w484
              n164 = Not(x=w489) -> (.not. x?=w488:bool)
              "MWhat?" <- w488
              n165 = call "SimLIDARPlot.vi"("data array [mag, phase (deg)]"=w485) -> ("SONAR"=→"ManualModeMapDAR":picture)  [unwired: 1 in]
              n166 = case shown="True" w484 {
                frame False {
                  # "No \nBeep"
                }
                frame True {
                  n167 = call <vilib>:"Beep.vi"("use system alert? (T)"=TRUE, "duration (msec)"=u32 1000, "frequency (Hz)"=u32 900) -> ()  [unwired: 9 in]
                }
              }
              n168 = Wait Until Next ms Multiple(millisecond multiple=u32 100 ("milliseconds to wait")) -> ()  [unwired: 1 out]
            }
            n169 = while {
              shift-right: [w513] -> _
              shift-left: _ -> [w512]
              stop <- w511 stop-if-true
              # "HowAmI?"
              n170 = local read "Battery\nVolts"() -> (w510:i16)
              n171 = local read "ManualModeStop"() -> (w511:bool)
              n172 = Not(x=w512) -> (.not. x?=w513:bool)
              n173 = Divide(x=w510, y=i16 1000) -> (x/y=→"Battery":dbl)
              n174 = Wait Until Next ms Multiple(millisecond multiple=u32 100 ("milliseconds to wait")) -> ()  [unwired: 1 out]
              "How? 2" <- w512
            }
            n175 = while {
              shift-right: [w507] -> _
              shift-left: _ -> [w506]
              stop <- w505 stop-if-true
              # "ForebrainAct"
              n176 = local read "E-Stop"() -> (w503:bool)
              n177 = local read "ManualModeStop"() -> (w505:bool)
              n178 = Select(t=0.0, s=w503, f="Manual Vel") -> (s? t:f=w500:dbl)
              n179 = To Word Integer(number=w500) -> (16bit integer=w498:i16)
              "Speed" <- w498
              n180 = local read "Send String"() -> (→"Send String to NXT":string)
              n181 = To Word Integer(number="Behavior Command") -> (16bit integer=w495:i16)
              n182 = local write "Upper Midbrain Active"("Upper Midbrain Active") -> ()
              n183 = local write "Mode"(w495) -> ()
              n184 = local write "Desired \nVelocity"(w498) -> ()
              n185 = local write "Local\nHeading"("Manual Heading") -> ()
              n186 = Not(x=w506) -> (.not. x?=w507:bool)
              n187 = Wait Until Next ms Multiple(millisecond multiple=u32 50 ("milliseconds to wait")) -> ()  [unwired: 1 out]
              "ActManual" <- w506
            }
            n188 = local read "ManualModeStop"() -> (w456:bool)
            n189 = case shown="True" w456 {
              tunnel: [TRUE ("s") w517] -> w458
              tunnel: [T1."ManualMode" ("Tab") w518] -> w457
              frame False {
              }
              frame True {
                # "Debounce tab for clean transition"
                n190 = flat-sequence {
                  tunnel: [w524] -> w518
                  tunnel: [TRUE ("s")] -> w517
                  frame #0 {
                    n191 = Wait (ms)(milliseconds to wait=u32 100) -> ()  [unwired: 1 out]
                  }
                  frame #1 {
                    w524 = T1."Startup&Shutdown" ("Tab")
                    # "Turn off\nVelocity\non \nExit"
                    n192 = local write "ManualModeStop"(FALSE ("ManualModeStop")) -> ()
                    n193 = local write "Desired \nVelocity"(i16 0 ("Desired \nVelocity")) -> ()
                    n194 = local write "Local\nHeading"(i16 0 ("Local\nHeading")) -> ()
                    n195 = local write "Mode"(i16 0 ("Mode")) -> ()
                    n196 = local write "Tab"(w524) -> ()
                  }
                }
              }
            }
          }
          frame "AutoMode" {
            n197 = flat-sequence {
              tunnel: w532 -> [_]
              tunnel: [w535] -> w530
              tunnel: w529 -> [w535]
              tunnel: w528 -> [w534]
              tunnel: [w534] -> w527
              tunnel: w526 -> [_]
              tunnel: w530 -> [w542]
              tunnel: w527 -> [w540]
              tunnel: [w622] -> w533
              tunnel: [FALSE ("s")] -> w531
              frame #0 {
                # "Run Robot\nbased on\nmission\ndefinition\nfile"
                n198 = local write "AutoMissionMap"(w534) -> ()
                n199 = while {
                  shift-right: [w538] -> _
                  shift-left: _ -> [w537]
                  stop <- "RunAutoMode" continue-if-true
                  # "Wait for Run\nbutton press\nbefore\nturning on\nAutoMode\nCode"
                  n200 = Not(x=w537) -> (.not. x?=w538:bool)
                  n201 = Wait Until Next ms Multiple(millisecond multiple=u32 100 ("milliseconds to wait")) -> ()  [unwired: 1 out]
                  "Ready" <- w537
                }
              }
              frame #1 {
                n202 = while {
                  shift-right: [w588] -> _
                  shift-left: _ -> [w579]
                  tunnel: w542 -> [w583]
                  shift-right: [w581] -> _
                  shift-left: _ -> [w582]
                  tunnel: w540 -> [w574]
                  stop <- w578 stop-if-true
                  # "WhereAmI?"
                  n203 = local read "WhereAmI?FromBase"() -> (w573:T6)
                  n204 = Get Date/Time In Seconds "GetMiissionCurrentTime"() -> (seconds since 1Jan1904=w584:timestamp)
                  n205 = call "WhereForebrainPerception.vi"("Where? Midbrain"=w573) -> ("(xr,yr)"=w581:cluster{"X":dbl, "Y":dbl}, "Direction"=w567:dbl)  [unwired: 3 in, 2 out]
                  "Robot Position" <- w581
                  n206 = local read "RunAutoMode"() -> (w578:bool)
                  n207 = Greater Or Equal?(x=w567, y=181.0) -> (x >= y?=w571:bool)
                  n208 = To Double Precision Float(number=w584) -> (double precision float=w585:dbl)
                  n209 = Subtract(x=w585, y=w583) -> (x-y=w586:dbl)
                  n210 = Not(x=w579) -> (.not. x?=w588:bool)
                  n211 = call "DrawRobot.vi"("(xr,yr) old"=w582, "(xr,yr) new"=w581, "2D Picture"=w574) -> ("new picture"=→"AutoMissionMap":picture)
                  n212 = local read "SteerAngle"() -> (w576:dbl)
                  n213 = Divide(x=w586, y=60.0) -> (x/y=w580:dbl)
                  "MissionTimeAuto" <- w580
                  n214 = Subtract(x=w567, y=360.0) -> (x-y=w569:dbl)
                  n215 = Select(t=w569, s=w571, f=w567) -> (s? t:f=w568:dbl)
                  n216 = shared-variable "My Computer\\RobotBrainExLibrary.lvlib\\MissionTime"(w580) -> ()  [unwired: 1 in, 1 out]
                  n217 = Bundle("Direction"=w568, "SteerAngle"=w576) -> (→"A Heading":cluster{"Direction":dbl, "SteerAngle":dbl})  [unwired: 1 in]
                  n218 = Wait Until Next ms Multiple(millisecond multiple=u32 50 ("milliseconds to wait")) -> ()  [unwired: 1 out]
                  "Where?" <- w579
                }
                n219 = while {
                  shift-right: [w612] -> _
                  shift-left: _ -> [w611]
                  shift-right: [w595] -> _
                  shift-left: 0.0 ("SteerAngle") -> [w607]
                  stop <- w614 stop-if-true
                  # "needs to put out heading in local coordinates"
                  # "Think"
                  n220 = Not(x=w611) -> (.not. x?=w612:bool)
                  n221 = Or(x="Pause", y="E-Stop") -> (x .or. y?=w592:bool)
                  n222 = Not(x="Manual Override") -> (.not. x?=w590:bool)
                  n223 = local read "WhereAmI?FromBase"() -> (w610:T6)
                  n224 = local read "WhatAroundMeMap?"() -> (w609:cluster{"T":dbl, "Range":dbl, "Bearing":dbl}[])
                  n225 = And(x=w590, y=w592) -> (x .and. y?=w593:bool)
                  n226 = local read "MDF"() -> (w600:T4)
                  n227 = call "GotoWaypoint.vi"("InhibitIn"=w593, "CurrentSteerAngle"=w607, "WhatAroundMe? Clean"=w609, "WhereAmI? Clean"=w610, "MDF In"=w600) -> ("BehCom"=→"Current Behavior":T7, "MDF Out"=w602:T4, "ActCommand"=→"WayPointAct":dbl[], "Vel"=w596:dbl, "SteerAngle"=w595:dbl)  [unwired: 1 in, 1 out]
                  "SteerAngle" <- w595
                  "A Speed" <- w596
                  n228 = To Long Integer(number=w596) -> (32bit integer=w597:i32)
                  n229 = To Long Integer(number=w595) -> (32bit integer=w594:i32)
                  n230 = local write "MDF"(w602) -> ()
                  n231 = local write "Desired \nVelocity"(w597) -> ()
                  n232 = local read "RunAutoMode"() -> (w614:bool)
                  n233 = local write "Local\nHeading"(w594) -> ()
                  n234 = local read "MDF_Original"() -> (w605:T4)
                  n235 = local read "MDF"() -> (w604:T4)
                  n236 = Select(t=w605, s="Rerun MDF", f=w604) -> (s? t:f=w601:T4)
                  n237 = local write "MDF"(w601) -> ()
                  n238 = Wait Until Next ms Multiple(millisecond multiple=u32 50 ("milliseconds to wait")) -> ()  [unwired: 1 out]
                  "Neo-C" <- w611
                }
                n239 = while {
                  shift-right: [w560] -> _
                  shift-left: _ -> [w562]
                  stop <- w559 stop-if-true
                  # "WhatIsAroundMe?"
                  n240 = local read "WhatAroundMeMap?"() -> (w556:cluster{"T":dbl, "Range":dbl, "Bearing":dbl}[])
                  n241 = call "ProcessLidarData.vi"("WhatAroundMe?MM"=w556) -> ("Collision"=w557:bool, "data array [mag, phase (deg)]"=w561:cluster{"magnitude":dbl, "phase":dbl}[])
                  "CollisionLight 2" <- w557
                  n242 = local read "RunAutoMode"() -> (w559:bool)
                  n243 = call "SimLIDARPlot.vi"("data array [mag, phase (deg)]"=w561) -> ("SONAR"=→"AutoModeLIDAR":picture)  [unwired: 1 in]
                  n244 = Not(x=w562) -> (.not. x?=w560:bool)
                  "What?" <- w560
                  n245 = case shown="True" w557 {
                    frame False {
                      # "No \nBeep"
                    }
                    frame True {
                      n246 = call <vilib>:"Beep.vi"("use system alert? (T)"=TRUE, "duration (msec)"=u32 1000, "frequency (Hz)"=u32 900) -> ()  [unwired: 9 in]
                    }
                  }
                  n247 = Wait Until Next ms Multiple(millisecond multiple=u32 50 ("milliseconds to wait")) -> ()  [unwired: 1 out]
                }
                n248 = while {
                  shift-right: [w554] -> _
                  shift-left: _ -> [w553]
                  stop <- w552 stop-if-true
                  # "HowAmI?"
                  n249 = local read "Battery\nVolts"() -> (w550:i16)
                  n250 = local read "RunAutoMode"() -> (w552:bool)
                  n251 = Not(x=w553) -> (.not. x?=w554:bool)
                  n252 = Divide(x=w550, y=i16 1000) -> (x/y=→"AutoBattery":dbl)
                  n253 = Wait Until Next ms Multiple(millisecond multiple=u32 80 ("milliseconds to wait")) -> ()  [unwired: 1 out]
                  "How?" <- w553
                }
                n254 = while {
                  shift-right: [w547] -> _
                  shift-left: _ -> [w546]
                  stop <- w545 stop-if-true
                  # "calculate desired heading.vi"
                  # "see calc desired\nheading"
                  # "convert to \noutputtin\nDesired v and\nlocal heading"
                  # "chnage arbiter to be -180 to 180"
                  # "Note:\nadd other beh to\narbiter"
                  # "ForebrainAct"
                  n255 = local read "WayPointAct"() -> (w544:dbl[])
                  n256 = local read "RunAutoMode"() -> (w545:bool)
                  n257 = Not(x=w546) -> (.not. x?=w547:bool)
                  n258 = call "ForebrainArbiter.vi"("WaypointInput"=w544) -> ("ForebrainActCom"=w543:dbl[])  [unwired: 14 in]
                  n259 = shared-variable "My Computer\\RobotBrainExLibrary.lvlib\\ActCommand"(w543) -> ()  [unwired: 1 in, 1 out]
                  n260 = Wait Until Next ms Multiple(millisecond multiple=u32 50 ("milliseconds to wait")) -> ()  [unwired: 1 out]
                  "Act" <- w546
                }
              }
              frame #2 {
                w622 = T1."Startup&Shutdown" ("Tab")
                # "Set robot Vel to 0"
                # "Reset latched run\nswitch"
                # "Force control to\nShutdown Case"
                n261 = shared-variable "My Computer\\RobotBrainExLibrary.lvlib\\ForebrainCom"(T8 {"VelCom"=0.0, "BehCom"=enum."OpenFieldTransit"} ("ForebrainCom")) -> ()  [unwired: 1 in, 1 out]
                n262 = local write "RunAutoMode"(TRUE ("RunAutoMode")) -> ()
                n263 = Initialize Array(0.0 ("element"), 90 ("dimension size")) -> (w618:dbl[])
                n264 = shared-variable "My Computer\\RobotBrainExLibrary.lvlib\\ActCommand"(w618) -> ()  [unwired: 1 in, 1 out]
                n265 = shared-variable "My Computer\\RobotBrainExLibrary.lvlib\\Xstart"(200.0 ("Xstart")) -> ()  [unwired: 1 in, 1 out]
                n266 = shared-variable "My Computer\\RobotBrainExLibrary.lvlib\\Ystart"(400.0 ("Ystart")) -> ()  [unwired: 1 in, 1 out]
                n267 = local write "Tab"(w622) -> ()
              }
            }
          }
          frame "Documentation" {
            # "Add:\n1) Blinking lights in each loop to show that they are running"
            # "This mode is just a static data flow picture of the ForeBrain"
            n268 = Wait (ms)(milliseconds to wait=u32 500) -> ()  [unwired: 1 out]
          }
          frame "DebugTHINK" {
            w632 = T1."Startup&Shutdown" ("Tab")
            # "Add:\n1) a button for each midbrain behavior to help in debugging\n2) graph of \"neural\" arbiter brain waves for each actuator\n3) a button for each forebrain behavior"
            # "Put code here in place of delay"
            # "Sends Tab Control\nback to Startup\ncase"
            n269 = Wait (ms)(milliseconds to wait=u32 5000) -> ()  [unwired: 1 out]
            n270 = local write "Tab"(w632) -> ()
          }
        }
        n271 = Not(x=w212) -> (.not. x?=w195:bool)
        "Robot Live" <- w195
      }
      n272 = while {
        tunnel: w56 -> [w179]
        tunnel: w55 -> [w178]
        tunnel: [w177] -> w53
        tunnel: [w176] -> w54
        shift-right: [w170] -> _
        shift-left: _ -> [w169]
        stop <- w180 continue-if-true
        w182 = 250  # timeout
        # "Finds and displays tugs position"
        # "runs continuously till program stops"
        # "Comminications with Base Station"
        # "receive string"
        # "If time out, post timeout and\nremove the timeout error"
        # "Read data from the port."
        n273 = Wait Until Next ms Multiple(millisecond multiple=u32 1) -> ()  [unwired: 1 out]
        n274 = UDP Read(connection ID=w179, timeout ms (25000)=w182, 8:w178) -> (data out=w171:string, error out=w183:errorcluster, 3:w176:refnum<k16>)  [unwired: 1 in, 2 out]
        n275 = local write "Base Station data rec'd"(w171) -> ()
        n276 = Unbundle By Name(w183) -> ("code"=w186:i32)
        n277 = Equal?(x=w186, y=56) -> (x = y?=w184:bool)
        "BS Time Out?" <- w184
        n278 = case shown="True" w184 {
          tunnel: [w193 errorcluster {"status"=FALSE, "code"=0, "source"=""} ("error out")] -> w177
          tunnel: w183 -> [w193 _]
          frame False {
          }
          frame True {
          }
        }
        n279 = call "PC parse the data.vi"("Nav String"=w171, "Tug"="Tug letter") -> ("Buoy locations"=w175:cluster{"regular expression":string, i32, i32}[], "Tug Location"=w173:T13, "Valid?"=w174:bool)  [unwired: 1 out]
        "Valid ?" <- w174
        n280 = local write "Buoy locations"(w175) -> ()
        n281 = case shown="True" w174 {
          tunnel: w173 -> [_ w192]
          frame False {
            # "No \nchange"
          }
          frame True {
            # "New values from BaseStation"
            n282 = shared-variable "My Computer\\RobotBrainExLibrary.lvlib\\MissionTime"() -> (w191:dbl)  [unwired: 1 in, 1 out]
            n283 = Unbundle(w192) -> (w190:i32, w189:i32, w188:i32)  [unwired: 1 out]
            n284 = local write "Tug X"(w190) -> ()
            n285 = local write "Tug Y"(w189) -> ()
            n286 = local write "Tug H"(w188) -> ()
            n287 = Bundle(w191, w190, w189, w188) -> (w187:cluster{dbl, i32, i32, i32})  [unwired: 1 in]
            n288 = local write "WhereAmI?FromBase"(w187) -> ()
          }
        }
        n289 = local read "RunRobot"() -> (w180:bool)
        n290 = Not(x=w169) -> (.not. x?=w170:bool)
        "udp rate" <- w169
      }
      n291 = while {
        tunnel: w57 -> [_]
        stop <- w106 continue-if-true
        # "boat heading?"
        n292 = local read "Upper Midbrain Active"() -> (w105:bool)
        n293 = case shown="True" w105 {
          frame False {
            # "loop timimng \ncontrolled externally"
            # "Send commands to NXT"
            n294 = local read "Desired \nVelocity"() -> (w117:i16)
            n295 = local read "Local\nHeading"() -> (w116:i16)
            n296 = local read "Mode"() -> (w115:i16)
            n297 = case shown="2" w115 {
              tunnel: w117 -> [w120 w131 w138]
              tunnel: w116 -> [w119 w130 w139]
              tunnel: [w121 w126 w134] -> w109
              tunnel: i16 7 ("element") -> [w118 w127 w135]
              frame 0, Default {
                w122 = i16 0 ("element")
                n298 = Build Array(u8 91 ("element"), w118, w119, w120, i16 1 ("element"), w122, w122, w122, w122, w122, u8 93 ("element")) -> (w121:i16[])
              }
              frame 1 {
                w128 = i16 0 ("element")
                n299 = Build Array(u8 91 ("element"), w127, w130, w131, w128, i16 1 ("element"), w128, w128, w128, w128, u8 93 ("element")) -> (w126:i16[])
              }
              frame 2 {
                w136 = i16 0 ("element")
                n300 = Build Array(u8 91 ("element"), w135, w139, w138, w136, w136, i16 1 ("element"), w136, w136, w136, u8 93 ("element")) -> (w134:i16[])
              }
            }
            n301 = Select(t=u8[] [91, 7, 7, 7, 1, 0, 0, 0, 0, 0, 92], s="Soft E-Stop", f=w109) -> (s? t:f=w110:i16[])
            n302 = Add(x=w110, y=u8[] [0, 65, 65, 65, 65, 65, 65, 65, 65, 65, 0]) -> (x+y=w111:i16[])
            n303 = Byte Array To String(unsigned byte array=w111) -> (string=w108:string)
            n304 = local write "Send String"(w108) -> ()
          }
          frame True {
            # "tweakers"
            # "IR heading"
            n305 = local read "ManualModeStop"() -> (w156:bool)
            n306 = local read "Heading"() -> (w153:cluster{dbl, dbl})
            n307 = local read "Ir distance"() -> (w155:i16)
            n308 = local read "WhatAroundMeMap?"() -> (w154:cluster{"T":dbl, "Range":dbl, "Bearing":dbl}[])
            n309 = Bundle("Lider good scale mult"="Lider good scale mult", "Lider good scale add"="Lider good scale add", "Lider speed scale mult"="Lider speed scale mult", "Lider speed scale add"="Lider speed scale add", "Follow right?"="Follow right?", "IR Following Distance"="IR Following Distance", "IR scaling div"="IR scaling div", "Lidar cutoff"="Lidar cutoff") -> (w142:T14)  [unwired: 1 in]
            n310 = Unbundle(w153) -> (w152:dbl)  [unwired: 1 out]
            n311 = call "UpperMidbrain.vi"("Boat Heading"=w152, "tweak"=w142, "WhatAroundMeMap? 2"=w154, "SOFT E-STOP"=w156, "behavior weights"="behavior weights", "ir distance"=w155) -> ("string"=w157:string)  [unwired: 5 in]
            n312 = local write "Send String"(w157) -> ()
          }
        }
        n313 = local read "RunRobot"() -> (w106:bool)
      }
      n314 = while {
        tunnel: w57 -> [_]
        stop <- w76 continue-if-true
        # "Receive information from NXT"
        n315 = local read "String Received"() -> (w81:string)
        n316 = Wait Until Next ms Multiple(millisecond multiple=u32 100) -> ()  [unwired: 1 out]
        n317 = String Subset(string=w81, offset (0)=1, length (rest)=1 ("length (rest)")) -> (substring=w80:string)
        n318 = case shown="Default" w80 {
          tunnel: w81 -> [w88 w90]
          frame Default {
            n319 = Search/Split String(string=w88, search string/char (-)=",", offset (0)=1) -> (substring before match=w83:string)  [unwired: 2 out]
            n320 = Decimal String To Number(string=w83, offset=1) -> (number=w85:i32)  [unwired: 1 in, 1 out]
            n321 = To Word Integer(number=w85) -> (16bit integer=→"Ir distance":i16)
          }
          frame "N" {
            # "0-15"
            # "Parse command \"N\""
            n322 = String Subset(string=w90, offset (0)=2, length (rest)=4 ("length (rest)")) -> (substring=w101:string)
            n323 = String Subset(string=w90, offset (0)=6, length (rest)=3 ("length (rest)")) -> (substring=w97:string)
            n324 = String Subset(string=w90, offset (0)=9, length (rest)=2 ("length (rest)")) -> (substring=w93:string)
            n325 = Decimal String To Number(string=w101) -> (number=w104:i32)  [unwired: 2 in, 1 out]
            n326 = Decimal String To Number(string=w97) -> (number=w96:i32)  [unwired: 2 in, 1 out]
            n327 = Decimal String To Number(string=w93) -> (number=w94:i32)  [unwired: 2 in, 1 out]
            n328 = To Word Integer(number=w104) -> (16bit integer=w100:i16)
            n329 = To Word Integer(number=w96) -> (16bit integer=w95:i16)
            n330 = To Long Integer(number=w94) -> (32bit integer=w89:i32)
            n331 = local write "LidarDist"(w95) -> ()
            n332 = local write "Battery\nVolts"(w100) -> ()
            n333 = local write "IR Index"(w89) -> ()
          }
        }
        n334 = local read "RunRobot"() -> (w76:bool)
      }
      n335 = while {
        stop <- w75 continue-if-true
        # "Run Simulated MapDAR"
        n336 = local read "Tug X"() -> (w73:i32)
        n337 = local read "Tug Y"() -> (w72:i32)
        n338 = local read "Tug H"() -> (w71:i32)
        n339 = Bundle "Bundle"("Tug X"=w73, "Tug Y"=w72, "Tug H"=w71) -> (w74:cluster{"Tug X":i32, "Tug Y":i32, "Tug H":i32})  [unwired: 1 in]
        n340 = call "HindbrainLIDAR_Sim.vi"("SubPosition"=w74) -> ("WhatAroundMe?"=→"WhatAroundMeMap?":cluster{"T":dbl, "Range":dbl, "Bearing":dbl}[])  [unwired: 10 in]
        n341 = local read "RunRobot"() -> (w75:bool)
      }
    }
    frame #2 {
      # "Close XBee Radio"
      # "Close UDP port"
      # "Realease LIDAR\nMemory"
      # "Reset Run \nSwitch"
      # "Shutdown Robot"
      n342 = call "Pixel_LIDAR_Close.vi"("error in (no error) 2"=w638, "Image"=w639) -> ()  [unwired: 1 in]
      n343 = local write "RunRobot"(TRUE ("RunRobot")) -> ()
      n344 = call "XB PC Close.vi"("error in (no error)"=w636, "VISA resource name"=w637) -> ()
      n345 = UDP Close(connection ID=w635, 8:w634) -> ()  [unwired: 2 out]
      "error out" <- w636
    }
  }
